vi "Polar to Cartesian FPGA simulator.vi"() -> ()   [LabVIEW 2015]
panel:
  out "Final Position":cluster{"X":dbl, "Y":dbl}={"X"=174.10813759359596, "Y"=984.7265389049335}
  out "Before ofset":cluster{dbl, dbl}={174.10813759359596, 984.7265389049335}
  out "before radius":cluster{dbl, dbl}={0.17410813759359595, 0.9847265389049334}
  out "Selected Element":u32=175
  out "XY Graph":cluster{"X":dbl, "Y":dbl}[](graph)
  out "y":dbl=173.64817766693034
  out "x":dbl=984.8077530122081
  out "r * e^(i*theta)":cdb=984.8077530122081+173.64817766693034i
  in  "Angle":dbl=10.0
  in  "Radius":dbl=1000.0
  in  "Y Center":dbl
  in  "X Center":dbl
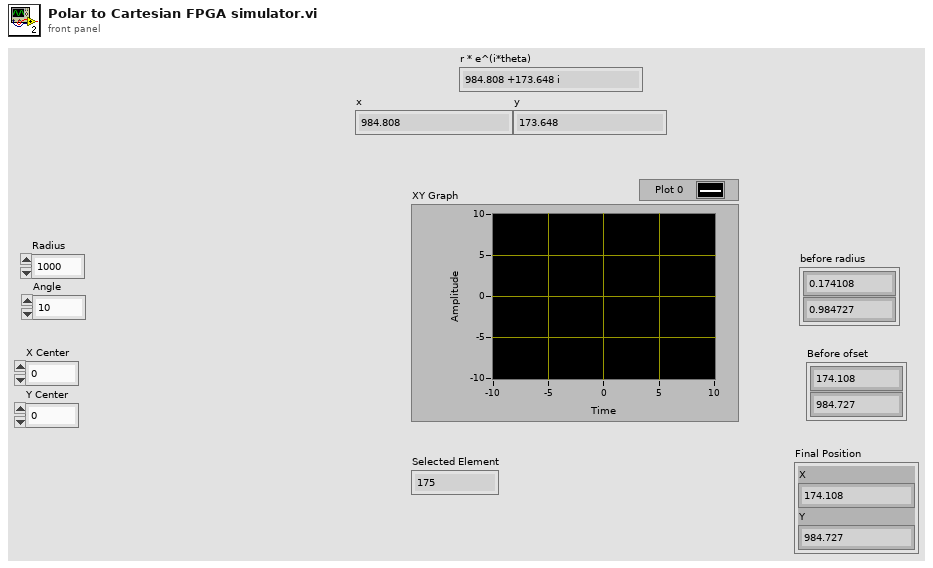
[diagram p1: front panel]
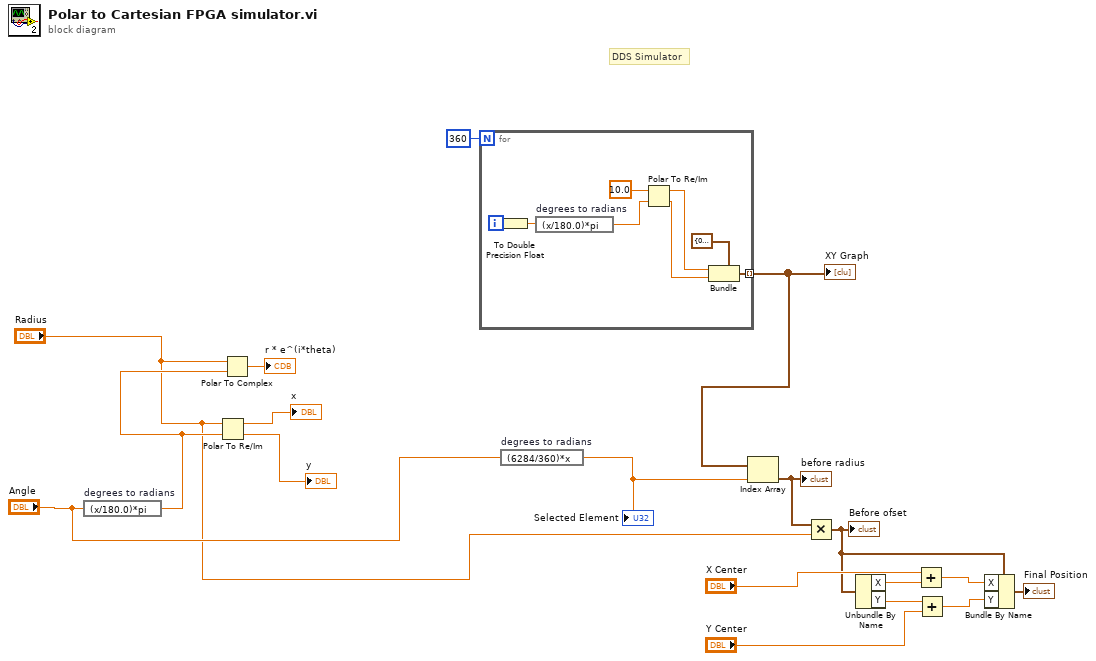
[diagram p0: block diagram]
diagram:
  # "DDS Simulator"
  n1 = expression code="(x/180.0)*pi" "degrees to radians"("Angle") -> (w15:dbl)
  n2 = Polar To Re/Im(2:w15, 3:"Radius") -> (0:→"y":dbl, 1:→"x":dbl)
  n3 = Polar To Complex(1:w15, 2:"Radius") -> (0:→"r * e^(i*theta)":cdb)
  n4 = for {
    N: 360 -> [_]
    tunnel: [w26] -> w14 mode=indexing
    i -> [w24]
    n5 = To Double Precision Float(number=w24) -> (double precision float=w23:dbl)
    n6 = expression code="(x/180.0)*pi" "degrees to radians"(w23) -> (w22:dbl)
    n7 = Polar To Re/Im(2:w22, 3:10.0 ("r")) -> (0:w19:dbl, 1:w20:dbl)
    n8 = Bundle(cluster=cluster{"X":dbl, "Y":dbl} {"X"=0.0, "Y"=0.0}, "X"=w20, "Y"=w19) -> (w26:cluster{"X":dbl, "Y":dbl})
  }
  "XY Graph" <- w14
  n9 = expression code="(6284/360)*x" "degrees to radians"("Angle") -> (w12:dbl)
  "Selected Element" <- w12
  n10 = Index Array(array=w14, index=w12) -> (element=w11:cluster{"X":dbl, "Y":dbl})
  "before radius" <- w11
  n11 = Multiply(x=w11, y="Radius") -> (x*y=w5:cluster{"X":dbl, "Y":dbl})
  "Before ofset" <- w5
  n12 = Unbundle By Name(w5) -> ("X"=w8:dbl, "Y"=w7:dbl)
  n13 = Add(x="X Center", y=w8) -> (x+y=w4:dbl)
  n14 = Add(x=w7, y="Y Center") -> (x+y=w3:dbl)
  n15 = Bundle By Name(cluster=w5, "X"=w4, "Y"=w3) -> (→"Final Position":cluster{"X":dbl, "Y":dbl})
